vi "BAM Generation Connections List_Initialize.vi"(8 "error in (no error)":errorcluster) -> (0 "error out":errorcluster {"code" min=0 max=0}, 3 "BAM Gen":T1)   [LabVIEW 2015, in "J1939 Addon Engine.lvlib"]
uses:
  J1939 Addon Engine.lvlib
  Types/BAM Generation Connections List_Ref.ctl
  Types/BAM Generation Connection Cluster.ctl
  Shared/J1939 Utilities/Types/CAN Outgoing Message Cluster.ctl
  Types/TP Connections List State.ctl
  Shared/J1939 Utilities/J1939 Utilities.lvlib
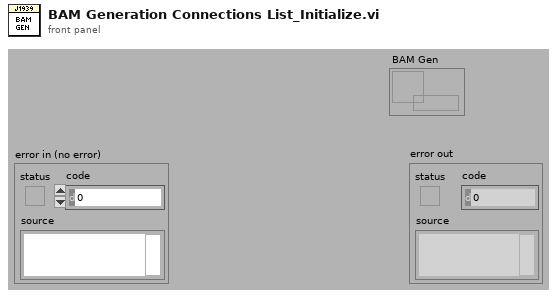
[diagram p1: front panel]
types:
  T1 = typedef "J1939 Addon Engine.lvlib/BAM Generation Connections List_Ref.ctl" = refnum<data-value>
  T2 = typedef "J1939 Addon Engine.lvlib/TP Connections List State.ctl" = enum16{"Add", "Update", "Get", "Remove", "Initialize"}
  T3 = typedef "J1939 Addon Engine.lvlib/BAM Generation Connection Cluster.ctl" = cluster{"Total Packets":u8, "Current Packet to Generate":u8, "Packets":T4[], "Previous Time Stamp":u32, "Total Bytes":u16, "Source Address":u8}
  T4 = typedef "J1939 Addon Shared.lvlib/J1939 Utilities.lvlib/CAN Outgoing Message Cluster.ctl" = cluster{"Identifier":u32, "Data":u8[]}
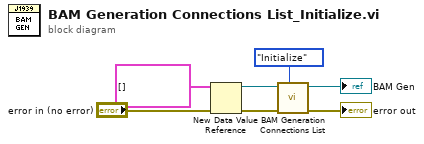
[diagram p0: block diagram]
diagram:
  n1 = New Data Value Reference(data value=T3[] [], error in="error in (no error)") -> (data value reference=w3:refnum<data-value>, error out=w5:errorcluster)
  n2 = call "BAM Generation Connections List.vi"("State"=TP_Connections_List_State."Initialize", "error in (no error)"=w5, "BAM Gen"=w3) -> ("error out"=→"error out":errorcluster, "BAM Gen out"=→"BAM Gen":T1)  [unwired: 5 in, 2 out]
